vi "VI Tree.vi"   [LabVIEW 2012, in "Keysight B2980 Series.lvlib"]
doc: "This is the instrument driver for the Keysignt B2980 Series Femto/Picoammeter/Electrometer/High Resistance Meter. The VI Tree displays all the user-callable VIs of the instrument driver in an organized table."
uses:
  Keysight B2980 Series.lvlib
  Data/Read Measurement (Multiple Point).vi
  Data/Low Level/Fetch Measurement (Multiple Point).vi
  Configure/Measurement/Configure Charge Measurement (Aperture).vi
  Configure/Measurement/Configure Current Measurement (Aperture).vi
  Configure/Measurement/Configure Resistance Measurement (Aperture).vi
  Configure/Measurement/Configure Voltage Measurement (Aperture).vi
panel:
  # "(c) 2014 National Instruments.  ALL RIGHTS RESERVED."
  # "SEE DIAGRAM\nFOR VI TREE."
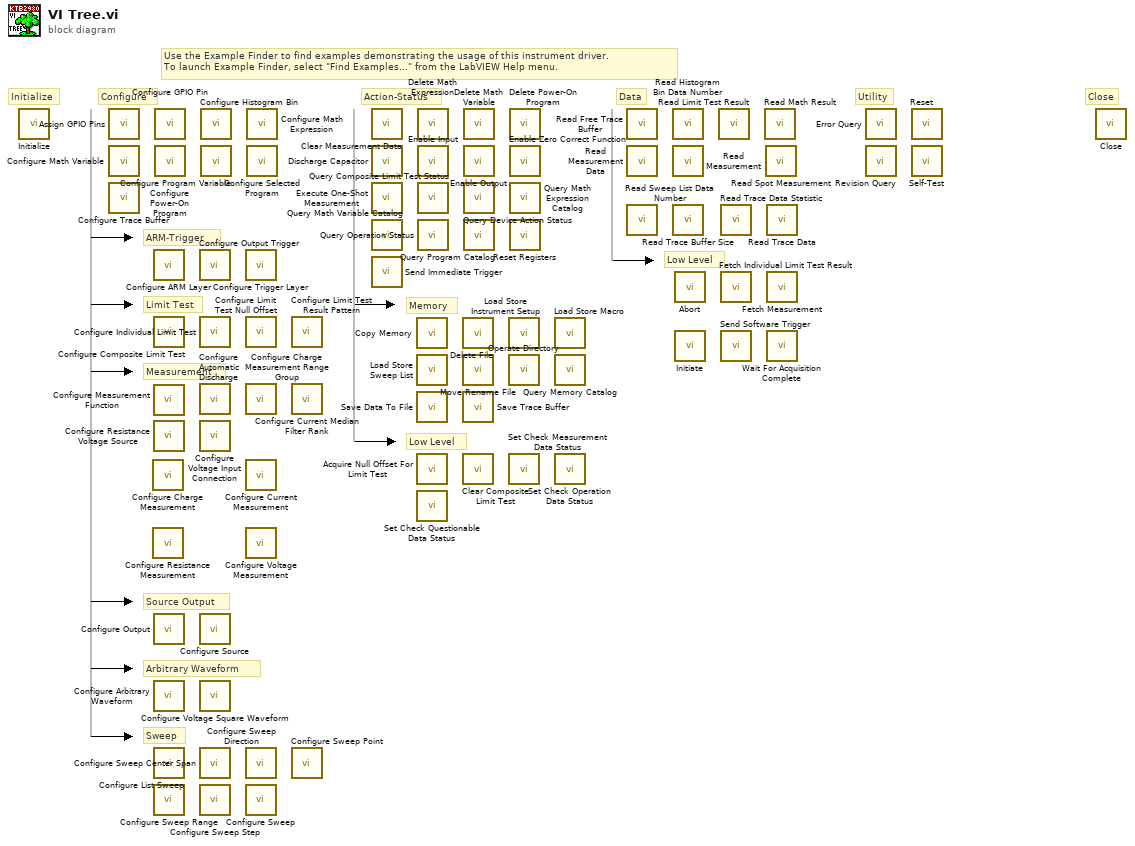
[diagram p0: block diagram]
diagram:
  # "Close"
  # "Utility"
  # "Low Level"
  # "Data"
  # "Sweep"
  # "Arbitrary Waveform"
  # "Source Output"
  # "Measurement"
  # "Limit Test"
  # "ARM-Trigger"
  # "Configure"
  # "Memory"
  # "Low Level"
  # "Action-Status"
  # "Initialize"
  # "Use the Example Finder to find examples demonstrating the usage of this instrument driver.\nTo launch Example Finder, select \"Find Examples...\" from the LabVIEW Help menu."
  n1 = call "Initialize.vi"() -> ()  [unwired: 10 in, 2 out]
  n2 = call "Assign GPIO Pins.vi"() -> ()  [unwired: 10 in, 2 out]
  n3 = call "Configure Math Variable.vi"() -> ()  [unwired: 10 in, 2 out]
  n4 = call "Configure Trace Buffer.vi"() -> ()  [unwired: 10 in, 2 out]
  n5 = call-poly "Configure Charge Measurement.vi"() -> ()  [unwired: 10 in, 2 out]
  n6 = call-poly "Configure Resistance Measurement.vi"() -> ()  [unwired: 10 in, 2 out]
  n7 = call "Configure ARM Layer.vi"() -> ()  [unwired: 14 in, 2 out]
  n8 = call "Configure Composite Limit Test.vi"() -> ()  [unwired: 14 in, 2 out]
  n9 = call "Configure Measurement Function.vi"() -> ()  [unwired: 10 in, 2 out]
  n10 = call "Configure Resistance Voltage Source.vi"() -> ()  [unwired: 10 in, 2 out]
  n11 = call "Configure Output.vi"() -> ()  [unwired: 10 in, 2 out]
  n12 = call "Configure Arbitrary Waveform.vi"() -> ()  [unwired: 10 in, 2 out]
  n13 = call "Configure List Sweep.vi"() -> ()  [unwired: 10 in, 2 out]
  n14 = call "Configure Sweep Range.vi"() -> ()  [unwired: 10 in, 2 out]
  n15 = call "Configure GPIO Pin.vi"() -> ()  [unwired: 14 in, 2 out]
  n16 = call "Configure Power-On Program.vi"() -> ()  [unwired: 10 in, 2 out]
  n17 = call "Configure Output Trigger.vi"() -> ()  [unwired: 14 in, 2 out]
  n18 = call "Configure Individual Limit Test.vi"() -> ()  [unwired: 14 in, 2 out]
  n19 = call "Configure Automatic Discharge.vi"() -> ()  [unwired: 10 in, 2 out]
  n20 = call "Configure Voltage Input Connection.vi"() -> ()  [unwired: 10 in, 2 out]
  n21 = call "Configure Source.vi"() -> ()  [unwired: 14 in, 2 out]
  n22 = call "Configure Voltage Square Waveform.vi"() -> ()  [unwired: 14 in, 2 out]
  n23 = call "Configure Sweep Center Span.vi"() -> ()  [unwired: 10 in, 2 out]
  n24 = call "Configure Sweep Step.vi"() -> ()  [unwired: 10 in, 2 out]
  n25 = call "Configure Histogram Bin.vi"() -> ()  [unwired: 10 in, 2 out]
  n26 = call "Configure Program Variable.vi"() -> ()  [unwired: 10 in, 2 out]
  n27 = call "Configure Trigger Layer.vi"() -> ()  [unwired: 14 in, 2 out]
  n28 = call "Configure Limit Test Null Offset.vi"() -> ()  [unwired: 10 in, 2 out]
  n29 = call "Configure Charge Measurement Range Group.vi"() -> ()  [unwired: 10 in, 2 out]
  n30 = call-poly "Configure Current Measurement.vi"() -> ()  [unwired: 10 in, 2 out]
  n31 = call-poly "Configure Voltage Measurement.vi"() -> ()  [unwired: 10 in, 2 out]
  n32 = call "Configure Sweep Direction.vi"() -> ()  [unwired: 10 in, 2 out]
  n33 = call "Configure Sweep.vi"() -> ()  [unwired: 14 in, 2 out]
  n34 = call "Configure Math Expression.vi"() -> ()  [unwired: 10 in, 2 out]
  n35 = call "Configure Selected Program.vi"() -> ()  [unwired: 10 in, 2 out]
  n36 = call "Configure Limit Test Result Pattern.vi"() -> ()  [unwired: 14 in, 2 out]
  n37 = call "Configure Current Median Filter Rank.vi"() -> ()  [unwired: 10 in, 2 out]
  n38 = call "Configure Sweep Point.vi"() -> ()  [unwired: 10 in, 2 out]
  n39 = call "Clear Measurement Data.vi"() -> ()  [unwired: 10 in, 2 out]
  n40 = call "Discharge Capacitor.vi"() -> ()  [unwired: 10 in, 2 out]
  n41 = call "Execute One-Shot Measurement.vi"() -> ()  [unwired: 10 in, 2 out]
  n42 = call "Query Math Variable Catalog.vi"() -> ()  [unwired: 9 in, 3 out]
  n43 = call "Send Immediate Trigger.vi"() -> ()  [unwired: 10 in, 2 out]
  n44 = call "Copy Memory.vi"() -> ()  [unwired: 10 in, 2 out]
  n45 = call "Load Store Sweep List.vi"() -> ()  [unwired: 10 in, 2 out]
  n46 = call "Save Data To File.vi"() -> ()  [unwired: 10 in, 2 out]
  n47 = call "Acquire Null Offset For Limit Test.vi"() -> ()  [unwired: 9 in, 3 out]
  n48 = call "Set Check Questionable Data Status.vi"() -> ()  [unwired: 9 in, 3 out]
  n49 = call "Delete Math Expression.vi"() -> ()  [unwired: 10 in, 2 out]
  n50 = call "Enable Input.vi"() -> ()  [unwired: 9 in, 3 out]
  n51 = call "Query Composite Limit Test Status.vi"() -> ()  [unwired: 9 in, 3 out]
  n52 = call "Query Operation Status.vi"() -> ()  [unwired: 8 in, 4 out]
  n53 = call "Delete File.vi"() -> ()  [unwired: 10 in, 2 out]
  n54 = call "Move Rename File.vi"() -> ()  [unwired: 10 in, 2 out]
  n55 = call "Save Trace Buffer.vi"() -> ()  [unwired: 10 in, 2 out]
  n56 = call "Clear Composite Limit Test.vi"() -> ()  [unwired: 10 in, 2 out]
  n57 = call "Delete Math Variable.vi"() -> ()  [unwired: 10 in, 2 out]
  n58 = call "Enable Output.vi"() -> ()  [unwired: 9 in, 3 out]
  n59 = call "Query Device Action Status.vi"() -> ()  [unwired: 9 in, 3 out]
  n60 = call "Query Program Catalog.vi"() -> ()  [unwired: 9 in, 3 out]
  n61 = call "Load Store Instrument Setup.vi"() -> ()  [unwired: 10 in, 2 out]
  n62 = call "Operate Directory.vi"() -> ()  [unwired: 10 in, 2 out]
  n63 = call "Set Check Measurement Data Status.vi"() -> ()  [unwired: 9 in, 3 out]
  n64 = call "Delete Power-On Program.vi"() -> ()  [unwired: 10 in, 2 out]
  n65 = call "Enable Zero Correct Function.vi"() -> ()  [unwired: 10 in, 2 out]
  n66 = call "Query Math Expression Catalog.vi"() -> ()  [unwired: 9 in, 3 out]
  n67 = call "Reset Registers.vi"() -> ()  [unwired: 10 in, 2 out]
  n68 = call "Load Store Macro.vi"() -> ()  [unwired: 10 in, 2 out]
  n69 = call "Query Memory Catalog.vi"() -> ()  [unwired: 9 in, 3 out]
  n70 = call "Set Check Operation Data Status.vi"() -> ()  [unwired: 9 in, 3 out]
  n71 = call "Read Free Trace Buffer.vi"() -> ()  [unwired: 8 in, 4 out]
  n72 = call "Read Measurement Data.vi"() -> ()  [unwired: 9 in, 3 out]
  n73 = call "Read Sweep List Data Number.vi"() -> ()  [unwired: 9 in, 3 out]
  n74 = call "Read Histogram Bin Data Number.vi"() -> ()  [unwired: 6 in, 6 out]
  n75 = call-poly "Read Measurement.vi"() -> ()  [unwired: 9 in, 3 out]
  n76 = call "Read Trace Buffer Size.vi"() -> ()  [unwired: 9 in, 3 out]
  n77 = call "Abort.vi"() -> ()  [unwired: 10 in, 2 out]
  n78 = call "Initiate.vi"() -> ()  [unwired: 10 in, 2 out]
  n79 = call "Read Limit Test Result.vi"() -> ()  [unwired: 8 in, 4 out]
  n80 = call "Read Trace Data Statistic.vi"() -> ()  [unwired: 9 in, 3 out]
  n81 = call "Fetch Individual Limit Test Result.vi"() -> ()  [unwired: 9 in, 3 out]
  n82 = call "Send Software Trigger.vi"() -> ()  [unwired: 10 in, 2 out]
  n83 = call "Read Math Result.vi"() -> ()  [unwired: 9 in, 3 out]
  n84 = call "Read Spot Measurement.vi"() -> ()  [unwired: 9 in, 3 out]
  n85 = call "Read Trace Data.vi"() -> ()  [unwired: 9 in, 3 out]
  n86 = call-poly "Fetch Measurement.vi"() -> ()  [unwired: 9 in, 3 out]
  n87 = call "Wait For Acquisition Complete.vi"() -> ()  [unwired: 10 in, 2 out]
  n88 = call "Error Query.vi"() -> ()  [unwired: 8 in, 4 out]
  n89 = call "Revision Query.vi"() -> ()  [unwired: 8 in, 4 out]
  n90 = call "Reset.vi"() -> ()  [unwired: 10 in, 2 out]
  n91 = call "Self-Test.vi"() -> ()  [unwired: 8 in, 4 out]
  n92 = call "Close.vi"() -> ()  [unwired: 11 in, 1 out]
